vi "Alp Error to Human Readable.vi"(1 "Input Error Cluster":T1) -> (0 "Output Error Description":string[](array[string]))   [LabVIEW 2013, in "alpD41.lvlib"]
uses:
  <userlib>/alpD41/alpD41.lvlib
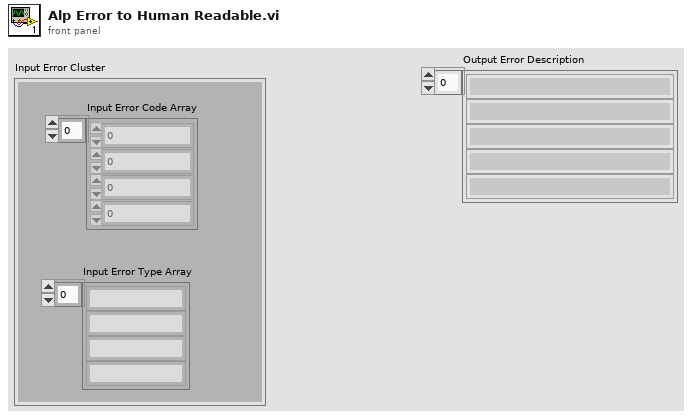
[diagram p1: front panel]
types:
  T1 = cluster{"Input Error Type Array":string[], "Input Error Code Array":dbl[]}
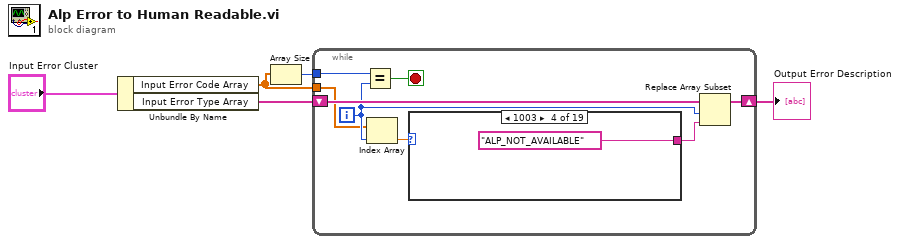
[diagram p0: block diagram]
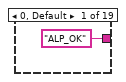
[diagram p2: hidden frame]
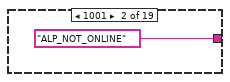
[diagram p3: hidden frame]
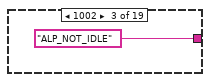
[diagram p4: hidden frame]
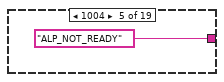
[diagram p5: hidden frame]
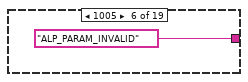
[diagram p6: hidden frame]
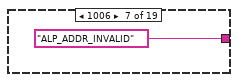
[diagram p7: hidden frame]
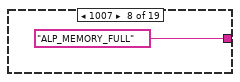
[diagram p8: hidden frame]
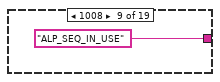
[diagram p9: hidden frame]
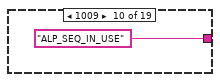
[diagram p10: hidden frame]
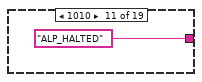
[diagram p11: hidden frame]
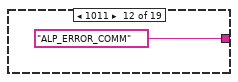
[diagram p12: hidden frame]
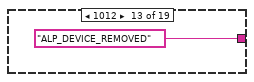
[diagram p13: hidden frame]
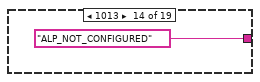
[diagram p14: hidden frame]
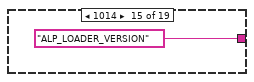
[diagram p15: hidden frame]
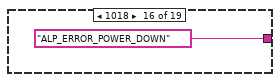
[diagram p16: hidden frame]
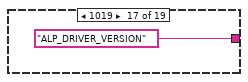
[diagram p17: hidden frame]
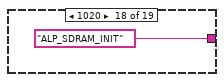
[diagram p18: hidden frame]
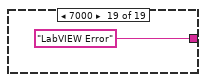
[diagram p19: hidden frame]
diagram:
  n1 = Unbundle By Name("Input Error Cluster") -> ("Input Error Code Array"=w3:dbl[], "Input Error Type Array"=w2:string[])
  n2 = Array Size(array=w3) -> (size(s)=w5:i32)
  n3 = while {
    tunnel: w5 -> [w12]
    tunnel: w3 -> [w6]
    shift-right: [w7] -> w1
    shift-left: w2 -> [w10]
    i -> [w8]
    stop <- w13 stop-if-true
    n4 = Equal?(x=w12, y=w8) -> (x = y?=w13:bool)
    n5 = Index Array(array=w6, index=w8) -> (element=w11:dbl)
    n6 = case shown="1003" w11 {
      tunnel: ["ALP_OK" "ALP_NOT_ONLINE" "ALP_NOT_IDLE" "ALP_NOT_AVAILABLE" "ALP_NOT_READY" "ALP_PARAM_INVALID" "ALP_ADDR_INVALID" "ALP_MEMORY_FULL" "ALP_SEQ_IN_USE" "ALP_SEQ_IN_USE" "ALP_HALTED" "ALP_ERROR_COMM" "ALP_DEVICE_REMOVED" "ALP_NOT_CONFIGURED" "ALP_LOADER_VERSION" "ALP_ERROR_POWER_DOWN" "ALP_DRIVER_VERSION" "ALP_SDRAM_INIT" "LabVIEW Error"] -> w9
      frame 0, Default {
      }
      frame 1001 {
      }
      frame 1002 {
      }
      frame 1003 {
      }
      frame 1004 {
      }
      frame 1005 {
      }
      frame 1006 {
      }
      frame 1007 {
      }
      frame 1008 {
      }
      frame 1009 {
      }
      frame 1010 {
      }
      frame 1011 {
      }
      frame 1012 {
      }
      frame 1013 {
      }
      frame 1014 {
      }
      frame 1018 {
      }
      frame 1019 {
      }
      frame 1020 {
      }
      frame 7000 {
      }
    }
    n7 = Replace Array Subset(array=w10, new element=w9, index=w8) -> (w7:string[])
  }
  "Output Error Description" <- w1
